vi "Find host address.vi"(0 "System number":i32=1 min=1 step=1, 1 "Port":i32=50000, 2 "Controller names":string[](array[string]), 3 "Mode":T1(ring), 5 "error in":errorcluster, 12 "Stop refnum":refnum<vi>) -> (14 "Address":string[](array[string]), 15 "ID":string[](array[string]), 16 "All Addresses":string[](array[string]), 17 "All IDs":string[](array[string]), 19 "error out":errorcluster)   [LabVIEW 2026]
doc: "Performs an UDP broadcast and returns IP addresses of all controllers matching Controller name. VI will also stop if Stop refnum or Local stop is TRUE.\n\nC-413: Controller names = C-413, Mode = Find XPort by UDP, Port = 30718\nC-413: Controller names = C-413, Mode = Find USR-K3 by UDP, Port = 1901\nC-702: Controller names = C-702, Mode = Find controller by UDP, Port = 50000\nC-867: Controller names = C-867, Mode = Find controller by UDP, Port = 50000\nC-884: Controller names = C-884, Mode = Find controller by UDP, Port = 50000\nC-885: Controller names = C-885, Mode = Find controller by UDP, Port = 50000\nC-886: Controller names = C-886, Mode = Find controller by UDP, Port = 50000\nC-891: Controller names = C-891, Mode = Find XPort by UDP, Port = 30718\nE-135: Controller names = E-135, Mode = Find USR-K3 by UDP, Port = 1901\nE-517: Controller names = E-517, Mode = Find controller by UDP, Port = 50000\nE-518: Controller names = E-518, Mode = Find controller by UDP, Port = 50000\nE-712: Controller names = E-712, Mode = Find controller by UDP, Port = 50000\nE-725: Controller names = E-725, Mode = Find XPort by UDP, Port = 30718\nE-727: Controller names = E-727, Mode = Find controller by UDP, Port = 50000\nE-753: Controller names = E-753, Mode = Find controller by UDP, Port = 50000\nE-754: Controller names = E-754, Mode = Find controller by UDP, Port = 50000\nE-871: Controller names = E-871, Mode = Find XPort by UDP, Port = 30718\nE-872: Controller names = E-872, Mode = Find controller by UDP, Port = 50000\nE-873: Controller names = E-873, Mode = Find XPort by UDP, Port = 30718\nE-874: Controller names = E-874, Mode = Find USR-K3 by UDP, Port = 1901\nF-206: Controller names = F-206, F-HEX, Mode = Find XPort by UDP, Port = 30718\nC-887, M-8X0: Controller names = M-8X0, HEXAPOD, Mode = Find XPort by UDP, Port = 30718"
uses:
  Available interfaces.ctl
  Global1.vi
  <vilib>/regexp/Match Regular Expression.xnode
panel:
  in  "stop":bool
  # "Performs an UDP broadcast and returns IP addresses of all controllers matching \"Controller name\"."
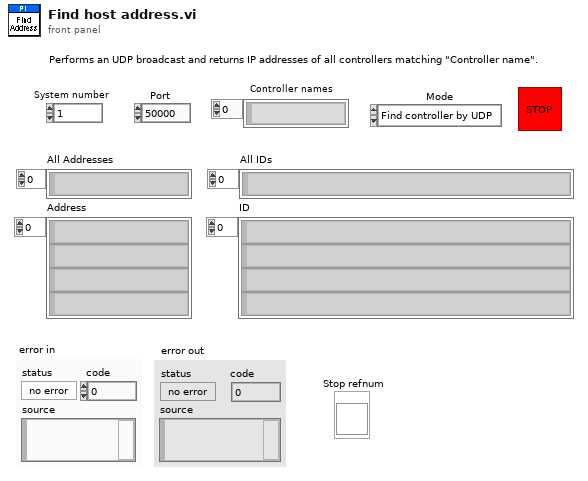
[diagram p1: front panel]
types:
  T1 = enum16{"Find controller by UDP", "Find XPort by UDP", "Find USR-K3 by UDP"}
  T2 = cluster{"Host address/name":string, "Port":i32, "Board":i32}
  T3 = typedef "Available interfaces.ctl" = u16
  T4 = cluster{"RS232 Portnumber":i32, "Timeout":i32, "RS232 Baud rate":u32, "Interface":T3, "GPIB Bus":i32, "GPIB Address":i32, "GPIB Mode":i32}
  T5 = cluster{"second":i32, "minute":i32, "hour":i32, "day of month":i32, "month":i32, "year":i32, "day of week":i32, "day of year":i32, "is DST":i32}
  T6 = cluster{"[0]":u8, "[1]":u8, "[2]":u8, "[3]":u8, "[4]":u8, "[5]":u8, "[6]":u8, "[7]":u8, "[8]":u8, "[9]":u8, "[10]":u8, "[11]":u8, "[12]":u8, "[13]":u8, "[14]":u8, "[15]":u8, "[16]":u8, "[17]":u8, "[18]":u8, "[19]":u8, "[20]":u8, "[21]":u8, "[22]":u8, "[23]":u8, "[24]":u8, "[25]":u8, "[26]":u8, "[27]":u8, "[28]":u8, "[29]":u8, "[30]":u8, "[31]":u8, "[32]":u8, "[33]":u8, "[34]":u8, "[35]":u8, "[36]":u8, "[37]":u8, "[38]":u8, "[39]":u8, "[40]":u8, "[41]":u8, "[42]":u8, "[43]":u8, "[44]":u8, "[45]":u8, "[46]":u8, "[47]":u8, "[48]":u8, "[49]":u8, "[50]":u8, "[51]":u8, "[52]":u8, "[53]":u8, "[54]":u8, "[55]":u8, "[56]":u8, "[57]":u8, "[58]":u8, "[59]":u8, "[60]":u8, "[61]":u8, "[62]":u8, "[63]":u8, "[64]":u8, "[65]":u8, "[66]":u8, "[67]":u8, "[68]":u8, "[69]":u8, "[70]":u8, "[71]":u8, "[72]":u8, "[73]":u8, "[74]":u8, "[75]":u8, "[76]":u8, "[77]":u8, "[78]":u8, "[79]":u8, "[80]":u8, "[81]":u8, "[82]":u8, "[83]":u8, "[84]":u8, "[85]":u8, "[86]":u8, "[87]":u8, "[88]":u8, "[89]":u8, "[90]":u8, "[91]":u8, "[92]":u8, "[93]":u8, "[94]":u8, "[95]":u8, "[96]":u8, "[97]":u8, "[98]":u8, "[99]":u8, "[100]":u8, "[101]":u8, "[102]":u8, "[103]":u8, "[104]":u8, "[105]":u8, "[106]":u8, "[107]":u8, "[108]":u8, "[109]":u8, "[110]":u8, "[111]":u8, "[112]":u8, "[113]":u8, "[114]":u8, "[115]":u8, "[116]":u8, "[117]":u8, "[118]":u8, "[119]":u8, "[120]":u8, "[121]":u8, "[122]":u8, "[123]":u8}
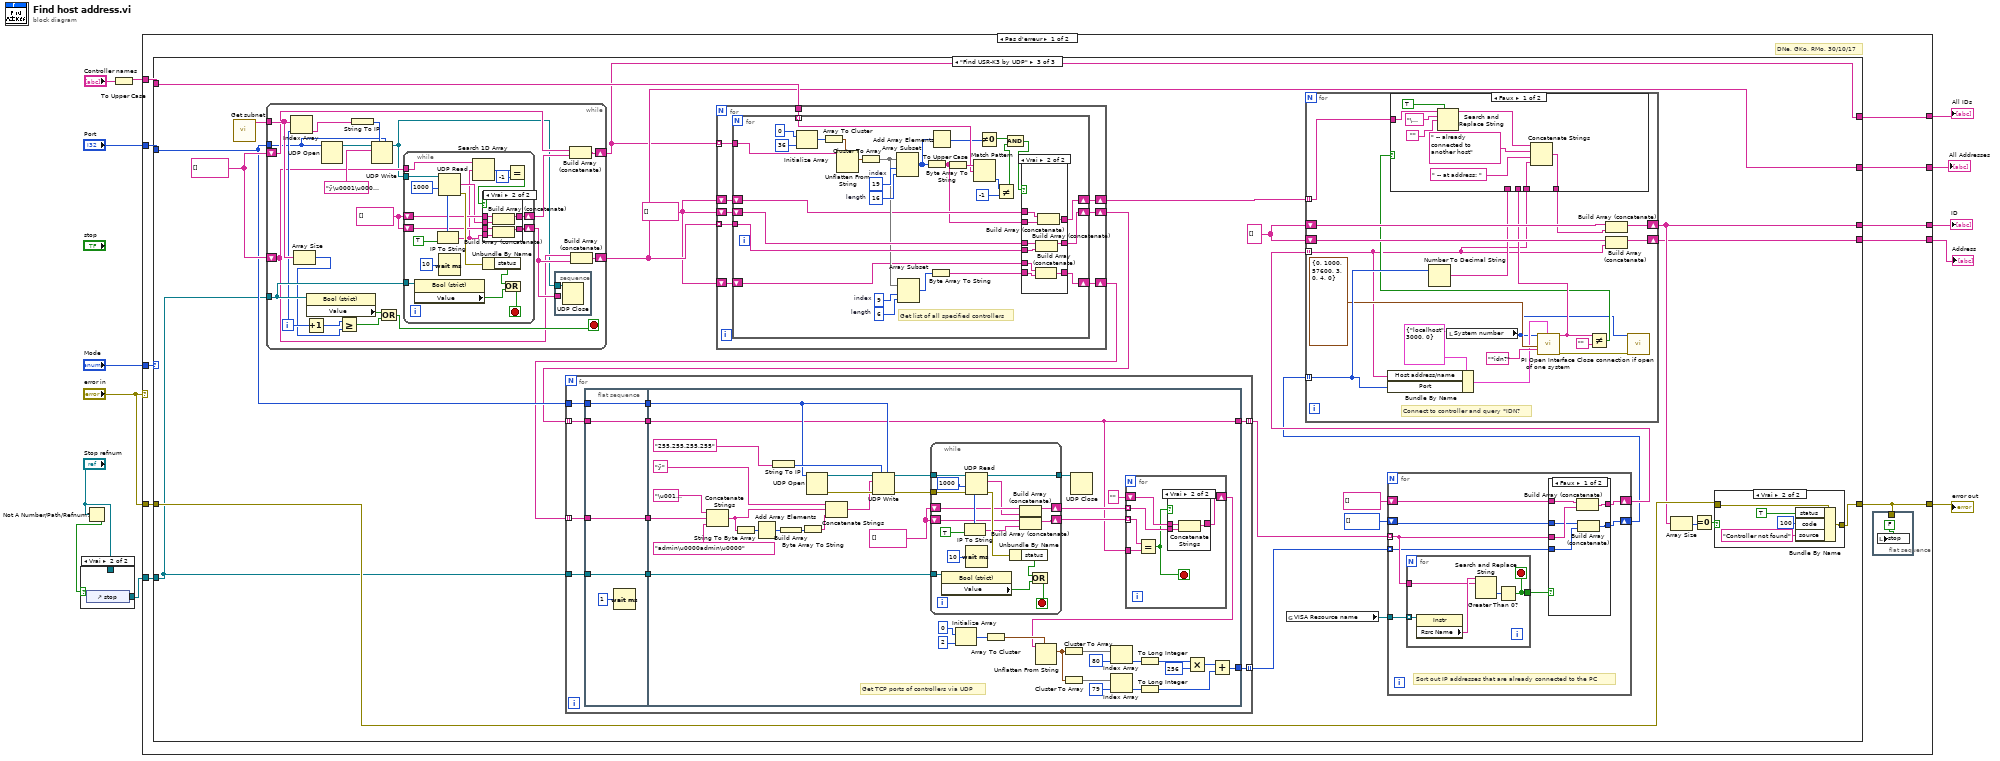
[diagram p0: block diagram]
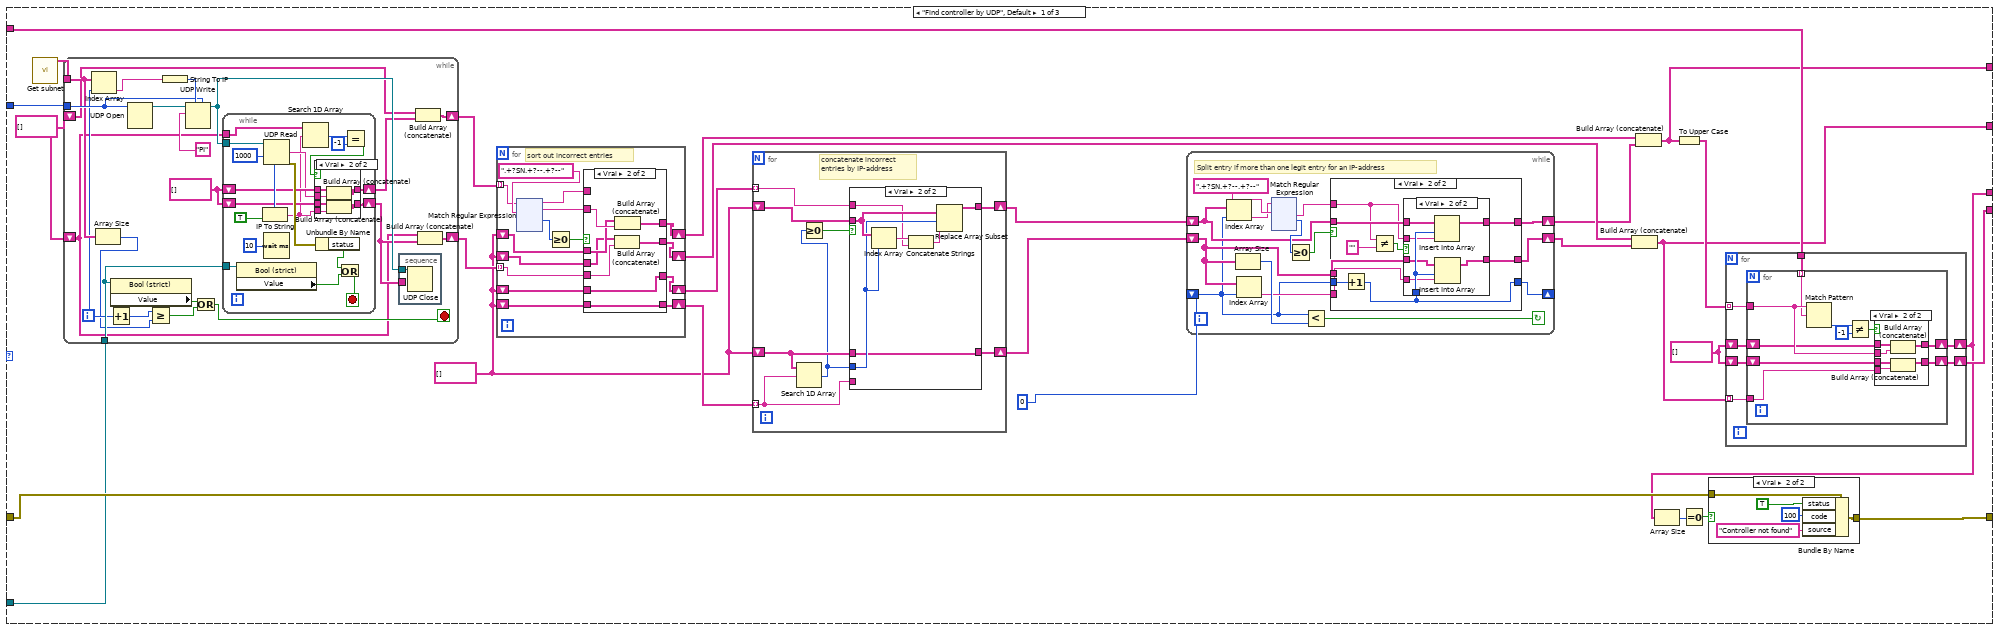
[diagram p3: hidden frame]
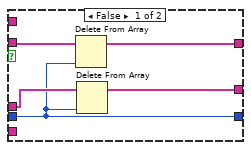
[diagram p4: hidden frame]
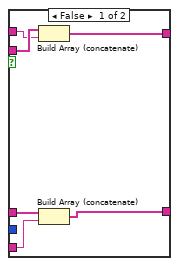
[diagram p6: hidden frame]
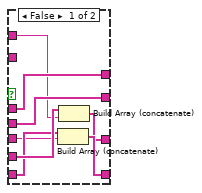
[diagram p7: hidden frame]
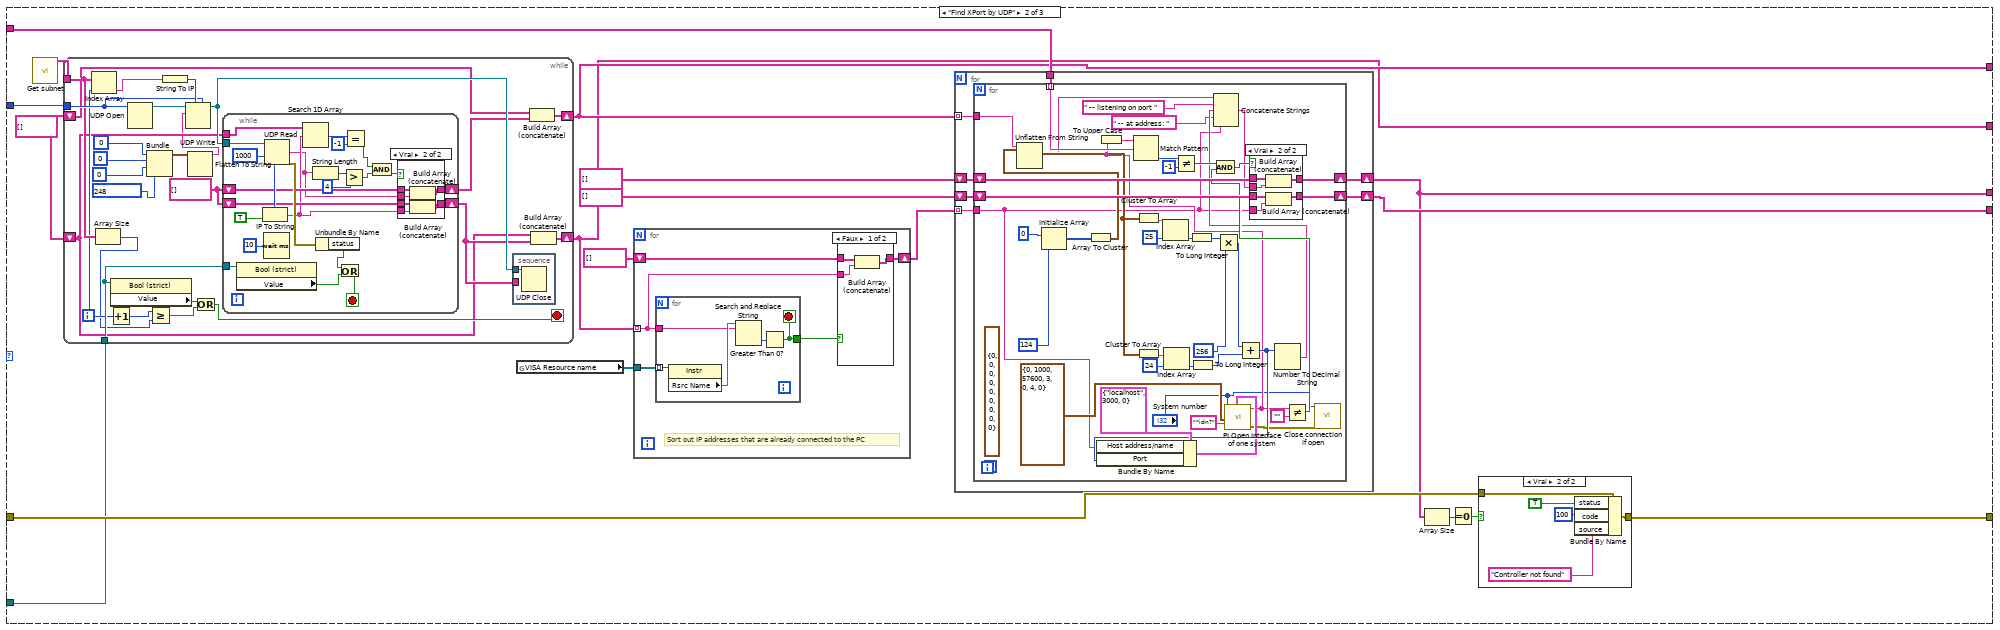
[diagram p11: hidden frame]
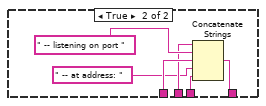
[diagram p17: hidden frame]
diagram:
  n1 = Not A Number/Path/Refnum?(number/path/refnum="Stop refnum") -> (NaN/Path/Refnum?=w7:bool)
  n2 = case shown="Vrai" w7 {
    tunnel: [w14 w15] -> w5
    tunnel: "Stop refnum" -> [w14 _]
    frame False {
    }
    frame True {
      n3 = control-ref of="stop"() -> (w15:refnum<vi>)
    }
  }
  n4 = To Upper Case(1:"Controller names") -> (0:w4:string[])
  n5 = case shown="Pas d'erreur" "error in" {
    tunnel: [w19 w886] -> w13
    tunnel: "error in" -> [w25 w886]
    tunnel: "Port" -> [w24 _]
    tunnel: "Mode" -> [w23 _]
    tunnel: w4 -> [w22 _]
    tunnel: [w21 string[] []] -> w2
    tunnel: [w17 string[] []] -> w9
    tunnel: [w18 string[] []] -> w8
    tunnel: w5 -> [w20 _]
    tunnel: [w16 string[] []] -> w1
    frame No Error {
      # "DNe, GKo, RMo, 30/10/17"
      n6 = case shown="\"Find USR-K3 by UDP\"" w23 {
        tunnel: w25 -> [w51 w472 w634]
        tunnel: [w50 w471 w633] -> w19
        tunnel: w24 -> [w49 w470 w627]
        tunnel: w22 -> [w40 w469 w632]
        tunnel: [w39 w463 w628] -> w21
        tunnel: [w48 w468 w623] -> w17
        tunnel: [w46 w466 w624] -> w18
        tunnel: w20 -> [w47 w467 w619]
        tunnel: [w36 w461 w629] -> w16
        frame "Find controller by UDP", Default {
          w28 = string[] []
          w44 = string[] []
          w27 = string[] []
          n7 = call "Get subnet.vi"() -> ("Subnet"=w45:string[])  [unwired: 19 out]
          n8 = while {
            tunnel: w49 -> [w395]
            tunnel: w47 -> [w392]
            tunnel: w45 -> [w393]
            shift-right: [w390] -> w41
            shift-left: w44 -> [w382]
            shift-right: [w384] -> w42
            shift-left: w44 -> [w378]
            i -> [w389]
            stop <- w386 stop-if-true
            w379 = string[] []
            n9 = Index Array(array=w393, index=w389) -> (element=w394:string)
            n10 = Array Size(array=w393) -> (size(s)=w385:i32)
            n11 = Increment(x=w389) -> (x+1=w388:i32)
            n12 = property class="Bool (strict)"(reference=w392) -> ("Value"=w391:bool)  [unwired: 1 in, 2 out]
            n13 = UDP Open(11:w395) -> (port=w398:refnum<k16>)  [unwired: 1 in, 5 out]
            n14 = Greater Or Equal?(x=w388, y=w385) -> (x >= y?=w387:bool)
            n15 = String To IP(1:w394) -> (0:w397:u32)
            n16 = UDP Write(address=w397, port or service name=w395, connection ID=w398, data in="PI") -> (3:w383:refnum<k16>)  [unwired: 1 in, 2 out]
            n17 = Or(x=w391, y=w387) -> (x .or. y?=w386:bool)
            n18 = while {
              tunnel: w383 -> [w419]
              tunnel: w392 -> [w415]
              shift-right: [w405] -> w381
              shift-left: w379 -> [w407]
              shift-right: [w403] -> w380
              shift-left: w379 -> [w404]
              tunnel: w378 -> [w401]
              stop <- w411 stop-if-true
              n19 = property class="Bool (strict)"(reference=w415) -> ("Value"=w414:bool)  [unwired: 1 in, 2 out]
              n20 = UDP Read(connection ID=w419, timeout ms (25000)=1000) -> (data out=w406:string, error out=w413:errorcluster, 6:w418:u32)  [unwired: 1 in, 3 out]
              n21 = IP To String(1:TRUE ("dot notation? (F)"), 2:w418) -> (0:w402:string)
              n22 = Wait (ms)(milliseconds to wait=u32 10) -> ()  [unwired: 1 out]
              n23 = Search 1D Array(1D array=w401, element=w402) -> (index of element=w410:i32)  [unwired: 1 out]
              n24 = Unbundle By Name(w413) -> ("status"=w412:bool)
              n25 = Or(x=w412, y=w414) -> (x .or. y?=w411:bool)
              n26 = Equal?(x=w410, y=-1) -> (x = y?=w408:bool)
              n27 = case shown="Vrai" w408 {
                tunnel: w407 -> [w421 w427]
                tunnel: w406 -> [_ w422]
                tunnel: [w421 w426] -> w405
                tunnel: w404 -> [w420 w425]
                tunnel: [w420 w424] -> w403
                tunnel: w402 -> [_ w423]
                frame False {
                }
                frame True {
                  n28 = Build Array (concatenate)(w427, w422) -> (w426:string[])
                  n29 = Build Array (concatenate)(w425, w423) -> (w424:string[])
                }
              }
            }
            n30 = stacked-sequence {
              tunnel: w383 -> [w399]
              tunnel: w380 -> [_]
              frame #0 {
                n31 = UDP Close(connection ID=w399) -> ()  [unwired: 1 in, 2 out]
              }
            }
            n32 = Build Array (concatenate)(w382, w381) -> (w390:string[])
            n33 = Build Array (concatenate)(w378, w380) -> (w384:string[])
          }
          n34 = for {
            tunnel: w41 -> [w243] mode=indexing
            tunnel: w42 -> [w239] mode=indexing
            shift-right: [w240] -> w38
            shift-left: w28 -> [w241]
            shift-right: [w237] -> w37
            shift-left: w28 -> [w238]
            shift-right: [w232] -> w34
            shift-left: w28 -> [w233]
            shift-right: [w230] -> w35
            shift-left: w28 -> [w234]
            # "sort out incorrect entries"
            n35 = xnode "Match Regular Expression"("chaîne en entrée"=w243, "expression régulière"=".+?SN.+?--.+?--" ("regular expression")) -> ("avant la correspondance"=w231:string, "toute l'expression"=w242:string, "offset après correspondance"=w236:i32)  [unwired: 2 in, 4 out]
            n36 = Greater Or Equal To 0?(x=w236) -> (x >= 0?=w235:bool)
            n37 = case shown="Vrai" w235 {
              tunnel: w242 -> [_ w260]
              tunnel: w241 -> [w251 w259]
              tunnel: [w251 w258] -> w240
              tunnel: w239 -> [w248 w257]
              tunnel: w238 -> [w252 w256]
              tunnel: [w252 w255] -> w237
              tunnel: w234 -> [w250 w253]
              tunnel: w233 -> [w249 w254]
              tunnel: [w247 w254] -> w232
              tunnel: w231 -> [w246 _]
              tunnel: [w245 w253] -> w230
              frame False {
                n38 = Build Array (concatenate)(w249, w248) -> (w247:string[])
                n39 = Build Array (concatenate)(w250, w246) -> (w245:string[])
              }
              frame True {
                n40 = Build Array (concatenate)(w256, w257) -> (w255:string[])
                n41 = Build Array (concatenate)(w259, w260) -> (w258:string[])
              }
            }
          }
          n42 = for {
            tunnel: w35 -> [w213] mode=indexing
            tunnel: w34 -> [w212] mode=indexing
            shift-right: [w215] -> w33
            shift-left: w28 -> [w216]
            shift-right: [w214] -> w32
            shift-left: w28 -> [w211]
            # "concatenate incorrect\nentries by IP-address"
            n43 = Search 1D Array(1D array=w211, element=w212) -> (index of element=w209:i32)  [unwired: 1 out]
            n44 = Greater Or Equal To 0?(x=w209) -> (x >= 0?=w210:bool)
            n45 = case shown="Vrai" w210 {
              tunnel: w216 -> [w222 w229]
              tunnel: w211 -> [w221 w223]
              tunnel: [w220 w224] -> w215
              tunnel: [w219 w223] -> w214
              tunnel: w213 -> [w218 w226]
              tunnel: w212 -> [w217 _]
              tunnel: w209 -> [_ w228]
              frame False {
                n46 = Build Array (concatenate)(w222, w218) -> (w220:string[])
                n47 = Build Array (concatenate)(w221, w217) -> (w219:string[])
              }
              frame True {
                n48 = Index Array(array=w229, index=w228) -> (element=w227:string)
                n49 = Concatenate Strings(w227, w226) -> (w225:string)
                n50 = Replace Array Subset(array=w229, new element=w225, index=w228) -> (w224:string[])
              }
            }
          }
          n51 = while {
            shift-right: [w61] -> w30
            shift-left: w33 -> [w59]
            shift-right: [w60] -> w31
            shift-left: w32 -> [w58]
            shift-right: [w54] -> _
            shift-left: 0 -> [w55]
            stop <- w67 continue-if-true
            # "Split entry if more than one legit entry for an IP-address"
            n52 = Index Array(array=w59, index=w55) -> (element=w65:string)
            n53 = Array Size(array=w58) -> (size(s)=w62:i32)
            n54 = Index Array(array=w58, index=w55) -> (element=w57:string)
            n55 = xnode "Match Regular Expression"("chaîne en entrée"=w65, "expression régulière"=".+?SN.+?--.+?--" ("regular expression")) -> ("après la correspondance"=w56:string, "offset après correspondance"=w64:i32)  [unwired: 2 in, 5 out]
            n56 = Greater Or Equal To 0?(x=w64) -> (x >= 0?=w63:bool)
            n57 = Less?(x=w55, y=w62) -> (x < y?=w67:bool)
            n58 = case shown="Vrai" w63 {
              tunnel: w58 -> [w71 w81]
              tunnel: w55 -> [w68 w82]
              tunnel: [w69 w77] -> w61
              tunnel: [w72 w80] -> w60
              tunnel: w59 -> [w70 w79]
              tunnel: w56 -> [_ w75]
              tunnel: w57 -> [_ w78]
              tunnel: [w68 w73] -> w54
              frame False {
                n59 = Delete From Array(array=w70, index=w68) -> (array with subset deleted=w69:string[])  [unwired: 1 in, 1 out]
                n60 = Delete From Array(array=w71, index=w68) -> (array with subset deleted=w72:string[])  [unwired: 1 in, 1 out]
              }
              frame True {
                n61 = Increment(x=w82) -> (x+1=w73:i32)
                n62 = Not Equal?(x=w75, y="") -> (x != y?=w76:bool)
                n63 = case shown="Vrai" w76 {
                  tunnel: w73 -> [_ w91]
                  tunnel: w81 -> [w83 w90]
                  tunnel: [w83 w89] -> w80
                  tunnel: w79 -> [w84 w88]
                  tunnel: w75 -> [_ w87]
                  tunnel: w78 -> [_ w86]
                  tunnel: [w84 w85] -> w77
                  frame False {
                  }
                  frame True {
                    n64 = Insert Into Array(array=w88, index=w91, new element=w87) -> (w85:string[])
                    n65 = Insert Into Array(array=w90, index=w91, new element=w86) -> (w89:string[])
                  }
                }
              }
            }
          }
          n66 = Build Array (concatenate)(w37, w31) -> (w36:string[])
          n67 = Build Array (concatenate)(w38, w30) -> (w39:string[])
          n68 = To Upper Case(1:w39) -> (0:w43:string[])
          n69 = for {
            tunnel: w43 -> [w434] mode=indexing
            shift-right: [w433] -> w46
            shift-left: w27 -> [w430]
            shift-right: [w431] -> w48
            shift-left: w27 -> [w432]
            tunnel: w40 -> [w429]
            tunnel: w36 -> [w428] mode=indexing
            n70 = for {
              tunnel: w434 -> [w441]
              tunnel: w429 -> [w436] mode=indexing
              shift-right: [w440] -> w433
              shift-left: w430 -> [w437]
              shift-right: [w438] -> w431
              shift-left: w432 -> [w439]
              tunnel: w428 -> [w435]
              n71 = Match Pattern(string=w441, regular expression=w436) -> (offset past match=w444:i32)  [unwired: 4 out]
              n72 = Not Equal?(x=w444, y=-1) -> (x != y?=w442:bool)
              n73 = case shown="Vrai" w442 {
                tunnel: w441 -> [_ w448]
                tunnel: [w446 w450] -> w440
                tunnel: w439 -> [w445 w452]
                tunnel: [w445 w451] -> w438
                tunnel: w437 -> [w446 w449]
                tunnel: w435 -> [_ w447]
                frame False {
                }
                frame True {
                  n74 = Build Array (concatenate)(w449, w448) -> (w450:string[])
                  n75 = Build Array (concatenate)(w452, w447) -> (w451:string[])
                }
              }
            }
          }
          n76 = Array Size(array=w46) -> (size(s)=w53:i32)
          n77 = Equal To 0?(x=w53) -> (x = 0?=w52:bool)
          n78 = case shown="Vrai" w52 {
            tunnel: [w453 w455] -> w50
            tunnel: w51 -> [w453 w454]
            frame False {
            }
            frame True {
              n79 = Bundle By Name(cluster=w454, "status"=TRUE, "code"=100 ("Bundle Element"), "source"="Controller not found" ("Bundle Element")) -> (w455:errorcluster)
            }
          }
        }
        frame "Find XPort by UDP" {
          w464 = string[] []
          n80 = call "Get subnet.vi"() -> ("Subnet"=w465:string[])  [unwired: 19 out]
          n81 = while {
            tunnel: w470 -> [w514]
            tunnel: w467 -> [w511]
            tunnel: w465 -> [w512]
            shift-right: [w509] -> w463
            shift-left: w464 -> [w501]
            shift-right: [w503] -> w461
            shift-left: w464 -> [w497]
            i -> [w508]
            stop <- w505 stop-if-true
            w498 = string[] []
            n82 = Index Array(array=w512, index=w508) -> (element=w513:string)
            n83 = Array Size(array=w512) -> (size(s)=w504:i32)
            n84 = Increment(x=w508) -> (x+1=w507:i32)
            n85 = property class="Bool (strict)"(reference=w511) -> ("Value"=w510:bool)  [unwired: 1 in, 2 out]
            n86 = UDP Open(11:w514) -> (port=w516:refnum<k16>)  [unwired: 1 in, 5 out]
            n87 = Bundle(u8 0, u8 0, u8 0, u8 248) -> (w496:cluster{u8, u8, u8, u8})  [unwired: 1 out]
            n88 = Greater Or Equal?(x=w507, y=w504) -> (x >= y?=w506:bool)
            n89 = String To IP(1:w513) -> (0:w515:u32)
            n90 = Flatten To String(anything=w496) -> (data string=w491:string)  [unwired: 1 in, 4 out]
            n91 = UDP Write(address=w515, port or service name=w514, connection ID=w516, data in=w491) -> (3:w502:refnum<k16>)  [unwired: 1 in, 2 out]
            n92 = Or(x=w510, y=w506) -> (x .or. y?=w505:bool)
            n93 = while {
              tunnel: w502 -> [w541]
              tunnel: w511 -> [w537]
              shift-right: [w529] -> w500
              shift-left: w498 -> [w530]
              shift-right: [w527] -> w499
              shift-left: w498 -> [w528]
              tunnel: w497 -> [w525]
              stop <- w533 stop-if-true
              n94 = property class="Bool (strict)"(reference=w537) -> ("Value"=w536:bool)  [unwired: 1 in, 2 out]
              n95 = Wait (ms)(milliseconds to wait=u32 10) -> ()  [unwired: 1 out]
              n96 = UDP Read(connection ID=w541, timeout ms (25000)=1000) -> (data out=w524:string, error out=w535:errorcluster, 6:w540:u32)  [unwired: 1 in, 3 out]
              n97 = IP To String(1:TRUE ("dot notation? (F)"), 2:w540) -> (0:w526:string)
              n98 = Search 1D Array(1D array=w525, element=w526) -> (index of element=w532:i32)  [unwired: 1 out]
              n99 = String Length(string=w524) -> (length=w523:i32)
              n100 = Unbundle By Name(w535) -> ("status"=w534:bool)
              n101 = Or(x=w534, y=w536) -> (x .or. y?=w533:bool)
              n102 = Greater?(x=w523, y=4) -> (0:w521:bool)
              n103 = Equal?(x=w532, y=-1) -> (x = y?=w520:bool)
              n104 = And(x=w520, y=w521) -> (x .and. y?=w519:bool)
              n105 = case shown="Vrai" w519 {
                tunnel: w530 -> [w543 w549]
                tunnel: w524 -> [_ w544]
                tunnel: [w543 w548] -> w529
                tunnel: w528 -> [w542 w547]
                tunnel: [w542 w546] -> w527
                tunnel: w526 -> [_ w545]
                frame False {
                }
                frame True {
                  n106 = Build Array (concatenate)(w549, w544) -> (w548:string[])
                  n107 = Build Array (concatenate)(w547, w545) -> (w546:string[])
                }
              }
            }
            n108 = stacked-sequence {
              tunnel: w502 -> [w517]
              tunnel: w499 -> [_]
              frame #0 {
                n109 = UDP Close(connection ID=w517) -> ()  [unwired: 1 in, 2 out]
              }
            }
            n110 = Build Array (concatenate)(w501, w500) -> (w509:string[])
            n111 = Build Array (concatenate)(w497, w499) -> (w503:string[])
          }
          n112 = global read "Global1.vi" "VISA Resource name"() -> (w462:refnum<visa-resource-name>[])
          n113 = for {
            tunnel: w462 -> [w479]
            shift-right: [w477] -> w459
            shift-left: string[] [] -> [w480]
            tunnel: w461 -> [w478] mode=indexing
            # "Sort out IP addresses that are already connected to the PC"
            n114 = for {
              tunnel: w478 -> [w487]
              tunnel: [w490] -> w481
              tunnel: w479 -> [w489] mode=indexing
              stop <- w490 stop-if-true
              n115 = property class="Instr"(reference=w489) -> ("Rsrc Name"=w488:string)  [unwired: 1 in, 2 out]
              n116 = Search and Replace String(input string=w488, search string=w487) -> (offset past replacement=w486:i32)  [unwired: 1 in, 8 out]
              n117 = Greater Than 0?(x=w486) -> (x > 0?=w490:bool)
            }
            n118 = case shown="Faux" w481 {
              tunnel: w480 -> [w484 w485]
              tunnel: w478 -> [w483 _]
              tunnel: [w482 w485] -> w477
              frame False {
                n119 = Build Array (concatenate)(w484, w483) -> (w482:string[])
              }
              frame True {
              }
            }
          }
          n120 = for {
            shift-right: [w556] -> w466
            shift-left: string[] [] -> [w553]
            shift-right: [w554] -> w468
            shift-left: string[] [] -> [w555]
            tunnel: w469 -> [w552]
            tunnel: w459 -> [w551] mode=indexing
            tunnel: w463 -> [w550] mode=indexing
            n121 = for {
              tunnel: w552 -> [w591] mode=indexing
              shift-right: [w595] -> w556
              shift-left: w553 -> [w592]
              shift-right: [w593] -> w554
              shift-left: w555 -> [w594]
              tunnel: w551 -> [w559]
              tunnel: w550 -> [w561]
              (unwired) T5 {"second"=0, "minute"=0, "hour"=0, "day of month"=0, "month"=0, "year"=0, "day of week"=0, "day of year"=0, "is DST"=0} ("type")
              n122 = Initialize Array(u8 0 ("element"), 124 ("dimension size")) -> (w590:u8[])
              n123 = Array To Cluster(array=w590) -> (cluster=w577:T6)
              n124 = Unflatten From String(type=w577, binary string=w561) -> (value=w576:T6)  [unwired: 1 in, 4 out]
              n125 = Cluster To Array(cluster=w576) -> (array=w587:u8[])
              n126 = Cluster To Array(cluster=w576) -> (array=w580:u8[])
              n127 = Index Array(array=w587, index=25) -> (element=w585:u8)
              n128 = Index Array(array=w580, index=24) -> (element=w582:u8)
              n129 = To Long Integer(number=w585) -> (32bit integer=w584:i32)
              n130 = To Long Integer(number=w582) -> (32bit integer=w579:i32)
              n131 = Multiply(x=w584, y=256) -> (x*y=w578:i32)
              n132 = Add(x=w578, y=w579) -> (x+y=w572:i32)
              n133 = Bundle By Name(cluster=T2 {"Host address/name"="localhost", "Port"=3000, "Board"=0} ("TCP/IP\nConfiguration"), "Host address/name"=w559, "Port"=w572) -> (w571:T2)
              n134 = call "PI Open Interface of one system.vi"("System number"="System number", "Interface configuration"=T4 {"RS232 Portnumber"=0, "Timeout"=1000, "RS232 Baud rate"=57600, "Interface"=3, "GPIB Bus"=0, "GPIB Address"=4, "GPIB Mode"=0}, "String to Send"="*idn?", "TCP/IP\nConfiguration"=w571) -> ("String read"=w562:string, "error out"=w557:errorcluster)  [unwired: 8 in, 6 out]
              n135 = To Upper Case(1:w562) -> (0:w563:string)
              n136 = Match Pattern(string=w563, regular expression=w591) -> (offset past match=w597:i32)  [unwired: 4 out]
              n137 = Not Equal?(x=w597, y=-1) -> (x != y?=w569:bool)
              n138 = Number To Decimal String(number=w572) -> (decimal integer string=w564:string)  [unwired: 1 out]
              n139 = Concatenate Strings(w562, " -- listening on port " ("string"), w564, " -- at address: " ("string"), w559) -> (w566:string)
              n140 = Not Equal?(x=w562, y="") -> (x != y?=w567:bool)
              n141 = And(x=w569, y=w567) -> (x .and. y?=w568:bool)
              n142 = case shown="Vrai" w568 {
                tunnel: w566 -> [_ w601]
                tunnel: [w599 w603] -> w595
                tunnel: w594 -> [w598 w605]
                tunnel: [w598 w604] -> w593
                tunnel: w592 -> [w599 w602]
                tunnel: w559 -> [_ w600]
                frame False {
                }
                frame True {
                  n143 = Build Array (concatenate)(w602, w601) -> (w603:string[])
                  n144 = Build Array (concatenate)(w605, w600) -> (w604:string[])
                }
              }
              n145 = call "Close connection if open.vi"("System no."="System number", "error in"=w557) -> ()  [unwired: 1 in, 17 out]
            }
          }
          n146 = Array Size(array=w466) -> (size(s)=w474:i32)
          n147 = Equal To 0?(x=w474) -> (x = 0?=w473:bool)
          n148 = case shown="Vrai" w473 {
            tunnel: [w606 w608] -> w471
            tunnel: w472 -> [w606 w607]
            frame False {
            }
            frame True {
              n149 = Bundle By Name(cluster=w607, "status"=TRUE, "code"=100 ("Bundle Element"), "source"="Controller not found" ("Bundle Element")) -> (w608:errorcluster)
            }
          }
        }
        frame "Find USR-K3 by UDP" {
          w625 = string[] []
          w621 = string[] []
          w631 = string[] []
          n150 = call "Get subnet.vi"() -> ("Subnet"=w630:string[])  [unwired: 19 out]
          n151 = while {
            tunnel: w619 -> [w841]
            tunnel: w630 -> [w842]
            shift-right: [w839] -> w628
            shift-left: w631 -> [w832]
            shift-right: [w833] -> w629
            shift-left: w631 -> [w828]
            tunnel: w627 -> [w827]
            i -> [w838]
            stop <- w835 stop-if-true
            w829 = string[] []
            n152 = Index Array(array=w842, index=w838) -> (element=w843:string)
            n153 = Array Size(array=w842) -> (size(s)=w834:i32)
            n154 = Increment(x=w838) -> (x+1=w837:i32)
            n155 = property class="Bool (strict)"(reference=w841) -> ("Value"=w840:bool)  [unwired: 1 in, 2 out]
            n156 = UDP Open(11:w827) -> (port=w846:refnum<k16>)  [unwired: 1 in, 5 out]
            n157 = Greater Or Equal?(x=w837, y=w834) -> (x >= y?=w836:bool)
            n158 = String To IP(1:w843) -> (0:w845:u32)
            n159 = UDP Write(address=w845, port or service name=w827, connection ID=w846, data in="ÿ\u0001\u0001\u0002") -> (3:w826:refnum<k16>)  [unwired: 1 in, 2 out]
            n160 = Or(x=w840, y=w836) -> (x .or. y?=w835:bool)
            n161 = while {
              tunnel: w826 -> [w867]
              tunnel: w841 -> [w863]
              shift-right: [w853] -> w831
              shift-left: w829 -> [w855]
              shift-right: [w851] -> w830
              shift-left: w829 -> [w852]
              tunnel: w828 -> [w849]
              stop <- w859 stop-if-true
              n162 = property class="Bool (strict)"(reference=w863) -> ("Value"=w862:bool)  [unwired: 1 in, 2 out]
              n163 = UDP Read(connection ID=w867, timeout ms (25000)=1000) -> (data out=w854:string, error out=w861:errorcluster, 6:w866:u32)  [unwired: 1 in, 3 out]
              n164 = IP To String(1:TRUE ("dot notation? (F)"), 2:w866) -> (0:w850:string)
              n165 = Wait (ms)(milliseconds to wait=u32 10) -> ()  [unwired: 1 out]
              n166 = Search 1D Array(1D array=w849, element=w850) -> (index of element=w858:i32)  [unwired: 1 out]
              n167 = Unbundle By Name(w861) -> ("status"=w860:bool)
              n168 = Or(x=w860, y=w862) -> (x .or. y?=w859:bool)
              n169 = Equal?(x=w858, y=-1) -> (x = y?=w856:bool)
              n170 = case shown="Vrai" w856 {
                tunnel: w855 -> [w869 w875]
                tunnel: w854 -> [_ w870]
                tunnel: [w869 w874] -> w853
                tunnel: w852 -> [w868 w873]
                tunnel: [w868 w872] -> w851
                tunnel: w850 -> [_ w871]
                frame False {
                }
                frame True {
                  n171 = Build Array (concatenate)(w875, w870) -> (w874:string[])
                  n172 = Build Array (concatenate)(w873, w871) -> (w872:string[])
                }
              }
            }
            n173 = stacked-sequence {
              tunnel: w826 -> [w847]
              tunnel: w830 -> [_]
              frame #0 {
                n174 = UDP Close(connection ID=w847) -> ()  [unwired: 1 in, 2 out]
              }
            }
            n175 = Build Array (concatenate)(w832, w831) -> (w839:string[])
            n176 = Build Array (concatenate)(w828, w830) -> (w833:string[])
          }
          n177 = for {
            shift-right: [w782] -> w626
            shift-left: w621 -> [w783]
            tunnel: w632 -> [w781]
            tunnel: w629 -> [w780] mode=indexing
            tunnel: w628 -> [w779] mode=indexing
            shift-right: [w777] -> w622
            shift-left: w621 -> [w778]
            shift-right: [w775] -> w620
            shift-left: w621 -> [w776]
            n178 = for {
              tunnel: w781 -> [w804] mode=indexing
              shift-right: [w801] -> w782
              shift-left: w783 -> [w803]
              tunnel: w780 -> [w802]
              tunnel: w779 -> [w791]
              shift-right: [w796] -> w777
              shift-left: w778 -> [w795]
              shift-right: [w792] -> w775
              shift-left: w776 -> [w793]
              w800 = 6  # length
              w799 = 9  # index
              w812 = 16  # length
              w813 = 19  # index
              # "Get list of all specified controllers"
              n179 = Initialize Array(u8 0 ("element"), 36 ("dimension size")) -> (w809:u8[])
              n180 = Array To Cluster(array=w809) -> (cluster=w810:T6)
              n181 = Unflatten From String(type=w810, binary string=w791) -> (value=w811:T6)  [unwired: 1 in, 4 out]
              n182 = Cluster To Array(cluster=w811) -> (array=w798:u8[])
              n183 = Array Subset(array=w798, index=w813, length=w812) -> (w789:u8[])
              n184 = Array Subset(array=w798, index=w799, length=w800) -> (w797:u8[])
              n185 = Byte Array To String(unsigned byte array=w789) -> (string=w790:string)
              n186 = Byte Array To String(unsigned byte array=w797) -> (string=w794:string)
              n187 = Add Array Elements(numeric array=w789) -> (sum=w788:u8)
              n188 = To Upper Case(1:w790) -> (0:w806:string)
              n189 = Match Pattern(string=w806, regular expression=w804) -> (offset past match=w786:i32)  [unwired: 4 out]
              n190 = Not Equal To 0?(x=w788) -> (x != 0?=w787:bool)
              n191 = Not Equal?(x=w786, y=-1) -> (x != y?=w785:bool)
              n192 = And(x=w787, y=w785) -> (x .and. y?=w784:bool)
              n193 = case shown="Vrai" w784 {
                tunnel: [w816 w825] -> w801
                tunnel: w803 -> [w816 w824]
                tunnel: w802 -> [_ w823]
                tunnel: [w815 w822] -> w796
                tunnel: w794 -> [_ w821]
                tunnel: w795 -> [w815 w820]
                tunnel: w793 -> [w814 w819]
                tunnel: [w814 w818] -> w792
                tunnel: w790 -> [_ w817]
                frame False {
                }
                frame True {
                  n194 = Build Array (concatenate)(w820, w821) -> (w822:string[])
                  n195 = Build Array (concatenate)(w824, w823) -> (w825:string[])
                  n196 = Build Array (concatenate)(w819, w817) -> (w818:string[])
                }
              }
            }
          }
          n197 = for {
            tunnel: w627 -> [w698]
            tunnel: w626 -> [w696] mode=indexing
            tunnel: [w695] -> w615 mode=indexing
            tunnel: [w700] -> w616 mode=indexing
            tunnel: w622 -> [w699] mode=indexing
            tunnel: w619 -> [w697]
            n198 = flat-sequence {
              tunnel: w696 -> [w702]
              tunnel: w697 -> [w703]
              tunnel: w698 -> [w704]
              tunnel: w699 -> [w705]
              tunnel: [w705] -> w694
              tunnel: [w704] -> w693
              tunnel: [w703] -> w692
              tunnel: [w702] -> w691
              tunnel: [w729] -> w700
              tunnel: [w706] -> w695
              tunnel: w694 -> [w727]
              tunnel: w693 -> [w718]
              tunnel: w692 -> [w716]
              tunnel: w691 -> [w706]
              frame #0 {
                n199 = Wait (ms)(milliseconds to wait=u32 1) -> ()  [unwired: 1 out]
              }
              frame #1 {
                w714 = string[] []
                # "Get TCP ports of controllers via UDP"
                n200 = Concatenate Strings("\u0013\u0003" ("data in"), w727, "admin\u0000admin\u0000" ("data in")) -> (w721:string)
                n201 = String To Byte Array(string=w721) -> (unsigned byte array=w724:u8[])
                n202 = Add Array Elements(numeric array=w724) -> (sum=w723:u8)
                n203 = String To IP(1:"255.255.255.255" ("name")) -> (0:w719:u32)
                n204 = Build Array(w723) -> (w722:u8[])
                n205 = Byte Array To String(unsigned byte array=w722) -> (string=w720:string)
                n206 = UDP Open(11:w718) -> (port=w745:refnum<k16>, 0:w746:errorcluster)  [unwired: 1 in, 4 out]
                n207 = Concatenate Strings("ÿ" ("data in"), w721, w720) -> (w717:string)
                n208 = UDP Write(address=w719, port or service name=w718, connection ID=w745, data in=w717, 8:w746) -> (error out=w707:errorcluster, 3:w715:refnum<k16>)  [unwired: 1 out]
                n209 = while {
                  tunnel: w715 -> [w774]
                  tunnel: w716 -> [w770]
                  shift-right: [w763] -> w712
                  shift-left: w714 -> [w765]
                  shift-right: [w761] -> w711
                  shift-left: w714 -> [w762]
                  tunnel: [w758] -> w710
                  tunnel: w707 -> [w757]
                  stop <- w766 stop-if-true
                  n210 = property class="Bool (strict)"(reference=w770) -> ("Value"=w769:bool)  [unwired: 1 in, 2 out]
                  n211 = UDP Read(connection ID=w774, timeout ms (25000)=1000, 8:w757) -> (data out=w764:string, error out=w768:errorcluster, 3:w758:refnum<k16>, 6:w773:u32)  [unwired: 2 out]
                  n212 = IP To String(1:TRUE ("dot notation? (F)"), 2:w773) -> (0:w760:string)
                  n213 = Wait (ms)(milliseconds to wait=u32 10) -> ()  [unwired: 1 out]
                  n214 = Unbundle By Name(w768) -> ("status"=w767:bool)
                  n215 = Build Array (concatenate)(w765, w764) -> (w763:string[])
                  n216 = Build Array (concatenate)(w762, w760) -> (w761:string[])
                  n217 = Or(x=w767, y=w769) -> (x .or. y?=w766:bool)
                }
                n218 = Initialize Array(u8 0 ("element"), 2 ("dimension size")) -> (w743:u8[])
                n219 = Array To Cluster(array=w743) -> (cluster=w744:T6)
                n220 = UDP Close(connection ID=w710) -> ()  [unwired: 1 in, 2 out]
                n221 = for {
                  shift-right: [w750] -> w709
                  shift-left: "" -> [w751]
                  tunnel: w712 -> [w749] mode=indexing
                  tunnel: w711 -> [w748] mode=indexing
                  tunnel: w706 -> [w752]
                  stop <- w747 stop-if-true
                  n222 = Equal?(x=w748, y=w752) -> (x = y?=w747:bool)
                  n223 = case shown="Vrai" w747 {
                    tunnel: w751 -> [w753 w756]
                    tunnel: w749 -> [_ w755]
                    tunnel: [w753 w754] -> w750
                    frame False {
                    }
                    frame True {
                      n224 = Concatenate Strings(w756, w755) -> (w754:string)
                    }
                  }
                }
                n225 = Unflatten From String(type=w744, binary string=w709) -> (value=w731:T6)  [unwired: 1 in, 4 out]
                n226 = Cluster To Array(cluster=w731) -> (array=w730:u8[])
                n227 = Cluster To Array(cluster=w731) -> (array=w734:u8[])
                n228 = Index Array(array=w730, index=80) -> (element=w739:u8)
                n229 = Index Array(array=w734, index=79) -> (element=w736:u8)
                n230 = To Long Integer(number=w739) -> (32bit integer=w738:i32)
                n231 = To Long Integer(number=w736) -> (32bit integer=w733:i32)
                n232 = Multiply(x=w738, y=256) -> (x*y=w732:i32)
                n233 = Add(x=w732, y=w733) -> (x+y=w729:i32)
              }
            }
          }
          n234 = global read "Global1.vi" "VISA Resource name"() -> (w618:refnum<visa-resource-name>[])
          n235 = for {
            tunnel: w618 -> [w642]
            shift-right: [w640] -> w613
            shift-left: string[] [] -> [w643]
            tunnel: w615 -> [w641] mode=indexing
            tunnel: w616 -> [w639] mode=indexing
            shift-right: [w637] -> w612
            shift-left: i32[] [] -> [w638]
            # "Sort out IP addresses that are already connected to the PC"
            n236 = for {
              tunnel: w641 -> [w654]
              tunnel: [w657] -> w644
              tunnel: w642 -> [w656] mode=indexing
              stop <- w657 stop-if-true
              n237 = property class="Instr"(reference=w656) -> ("Rsrc Name"=w655:string)  [unwired: 1 in, 2 out]
              n238 = Search and Replace String(input string=w655, search string=w654) -> (offset past replacement=w653:i32)  [unwired: 1 in, 8 out]
              n239 = Greater Than 0?(x=w653) -> (x > 0?=w657:bool)
            }
            n240 = case shown="Faux" w644 {
              tunnel: w643 -> [w650 w652]
              tunnel: w641 -> [w649 _]
              tunnel: [w648 w652] -> w640
              tunnel: w639 -> [w645 _]
              tunnel: w638 -> [w647 w651]
              tunnel: [w646 w651] -> w637
              frame False {
                n241 = Build Array (concatenate)(w650, w649) -> (w648:string[])
                n242 = Build Array (concatenate)(w647, w645) -> (w646:i32[])
              }
              frame True {
              }
            }
          }
          n243 = for {
            shift-right: [w675] -> w624
            shift-left: w625 -> [w672]
            shift-right: [w673] -> w623
            shift-left: w625 -> [w674]
            tunnel: w613 -> [w661] mode=indexing
            tunnel: w612 -> [w671] mode=indexing
            tunnel: w620 -> [w660] mode=indexing
            # "Connect to controller and query *IDN?"
            n244 = Bundle By Name(cluster=T2 {"Host address/name"="localhost", "Port"=3000, "Board"=0} ("TCP/IP\nConfiguration"), "Host address/name"=w661, "Port"=w671) -> (w667:T2)
            n245 = Number To Decimal String(number=w671) -> (decimal integer string=w664:string)  [unwired: 1 out]
            n246 = local read "System number"() -> (w658:i32)
            n247 = call "PI Open Interface of one system.vi"("System number"=w658, "Interface configuration"=T4 {"RS232 Portnumber"=0, "Timeout"=1000, "RS232 Baud rate"=57600, "Interface"=3, "GPIB Bus"=0, "GPIB Address"=4, "GPIB Mode"=0}, "String to Send"="*idn?", "TCP/IP\nConfiguration"=w667) -> ("String read"=w663:string, "error out"=w659:errorcluster)  [unwired: 8 in, 6 out]
            n248 = Not Equal?(x=w663, y="") -> (x != y?=w662:bool)
            n249 = case shown="Faux" w662 {
              tunnel: [w684 w690] -> w665
              tunnel: w664 -> [_ w688]
              tunnel: w663 -> [_ w687]
              tunnel: w661 -> [w677 w685]
              tunnel: w660 -> [w683 _]
              frame False {
                n250 = Search and Replace String(replace all?=TRUE, input string=w683, search string="\u0000", replace string="") -> (result string=w679:string)  [unwired: 1 in, 6 out]
                n251 = Concatenate Strings(w679, " -- already connected to another host" ("string"), " -- at address: " ("string"), w677) -> (w684:string)
              }
              frame True {
                n252 = Concatenate Strings(w687, " -- listening on port " ("string"), w688, " -- at address: " ("string"), w685) -> (w690:string)
              }
            }
            n253 = Build Array (concatenate)(w672, w665) -> (w675:string[])
            n254 = Build Array (concatenate)(w674, w661) -> (w673:string[])
            n255 = call "Close connection if open.vi"("System no."=w658, "error in"=w659) -> ()  [unwired: 1 in, 17 out]
          }
          n256 = Array Size(array=w624) -> (size(s)=w636:i32)
          n257 = Equal To 0?(x=w636) -> (x = 0?=w635:bool)
          n258 = case shown="Vrai" w635 {
            tunnel: [w876 w878] -> w633
            tunnel: w634 -> [w876 w877]
            frame False {
            }
            frame True {
              n259 = Bundle By Name(cluster=w877, "status"=TRUE, "code"=100 ("Bundle Element"), "source"="Controller not found" ("Bundle Element")) -> (w878:errorcluster)
            }
          }
        }
      }
      n260 = flat-sequence {
        tunnel: w19 -> [_]
        frame #0 {
          n261 = local write "stop"(FALSE ("stop")) -> ()
        }
      }
    }
    frame Error {
    }
  }
  "error out" <- w13
  "Address" <- w9
  "ID" <- w8
  "All IDs" <- w2
  "All Addresses" <- w1
